vi "get_config_cluster.vi"(8 "error in (no error)":errorcluster, 11 "AnalyserDL090623TwoD in":refnum<class "AnalyserDL090623TwoD.lvclass">) -> (0 "error out":errorcluster, 2 "config cluster (variant)":variant, 3 "AnalyserDL090623TwoD out":refnum<class "AnalyserDL090623TwoD.lvclass">)   [LabVIEW 2010, in "AnalyserDL090623TwoD.lvclass"]
uses:
  AnalyserDL090623TwoD.lvclass
  AnalyserDL090623TwoD.lvclass/AnalyserDL090623TwoD.ctl
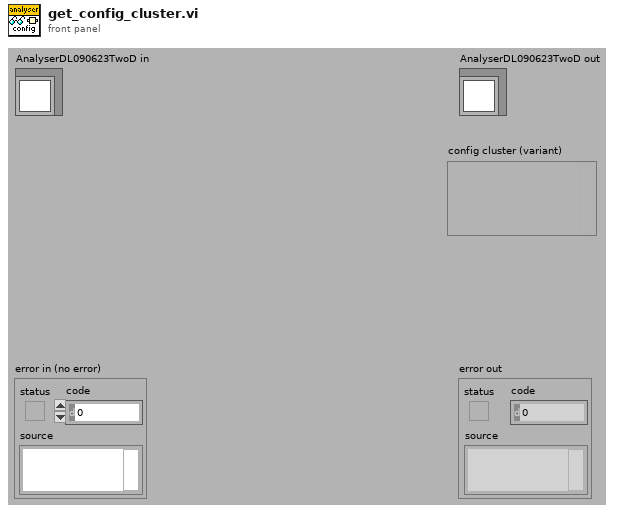
[diagram p1: front panel]
types:
  T1 = typedef "AnalyserDL090623TwoD.lvclass/config_data_cluster.ctl" = cluster{"segmenter":T2, "expression":string, "trace processor pipeline":T2[]}
  T2 = typedef "plugin_specification.ctl" = cluster{"class path":string, "configuration":string, "label":string, "settings name":string}
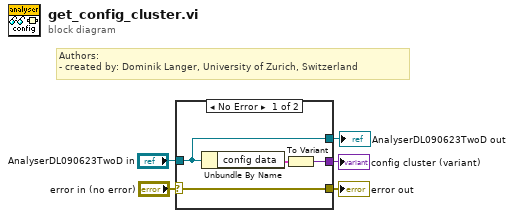
[diagram p0: block diagram]
diagram:
  # "Authors: \n- created by: Dominik Langer, University of Zurich, Switzerland"
  n1 = case shown="No Error" "error in (no error)" {
    selector: "error in (no error)" -> [w7 w11]
    tunnel: "AnalyserDL090623TwoD in" -> [w6 w10]
    tunnel: [w8 _] -> w3
    tunnel: [w7 w11] -> w1
    tunnel: [w6 w10] -> w2
    frame No Error {
      n2 = Unbundle By Name(w6) -> ("config data"=w9:T1)
      n3 = To Variant(anything=w9) -> (Variant=w8:variant)
    }
    frame Error {
    }
  }
  "error out" <- w1
  "AnalyserDL090623TwoD out" <- w2
  "config cluster (variant)" <- w3
